vi "MD5Checksum_string.vi"(11 "Message String":string) -> (2 "MD5 message-digest (Ascii)":string, 3 "MD5 message-digest (Hex)":string)   [LabVIEW 2016, in "vi_lib.lvlib"]
doc: "This VI computes the MD5 message-digest of a string, based on the algorithm described in RFC 1321 (http://www.ietf.org/rfc/rfc1321.txt). The MD5 message-digest is a 128-bit number, displayed in lower case hexadecimal."
uses:
  vi_lib.lvlib
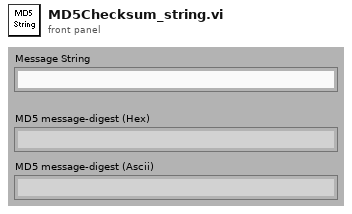
[diagram p1: front panel]
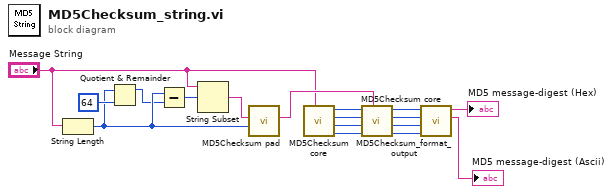
[diagram p0: block diagram]
diagram:
  n1 = String Length(string="Message String") -> (length=w5:i32)
  n2 = Quotient & Remainder(x=w5, y=64) -> (x-y*floor(x/y)=w4:i32)  [unwired: 1 out]
  n3 = Subtract(x=w5, y=w4) -> (x-y=w6:i32)
  n4 = String Subset(string="Message String", offset (0)=w6) -> (substring=w3:string)  [unwired: 1 out]
  n5 = call <vilib>:"MD5Checksum pad.vi"("Message String Length (bytes)"=w5, "Last Part of Message String"=w3) -> ("Padding"=w16:string)  [unwired: 9 out]
  n6 = call <vilib>:"MD5Checksum core.vi"("Input String"="Message String") -> ("s4 out"=w12:u32, "s3 out"=w13:u32, "s2 out"=w14:u32, "s1 out"=w15:u32)  [unwired: 4 in, 3 out]
  n7 = call <vilib>:"MD5Checksum core.vi"("Input String"=w16, "s4 in"=w12, "s3 in"=w13, "s2 in"=w14, "s1 in"=w15) -> ("s4 out"=w8:u32, "s3 out"=w9:u32, "s2 out"=w10:u32, "s1 out"=w11:u32)  [unwired: 3 out]
  n8 = call "MD5Checksum_format_output.vi"("s4"=w8, "s3"=w9, "s2"=w10, "s1"=w11) -> ("MD5 message-digest (ASCII)"=→"MD5 message-digest (Ascii)":string, "MD5 message-digest (HEX)"=→"MD5 message-digest (Hex)":string)  [unwired: 6 out]
